vi "Earthquake.vi"(11 "VI Ref":refnum<vi>) -> ()   [LabVIEW 2019]
doc: "Earthquake disaster. Violently shakes the block diagram left and right, with each object having a 20% chance of being destroyed."
uses:
  _Sound/Music Player Command Message.ctl
  _Sound/Music Player Command.ctl
  _Sound/Sound.lvlib
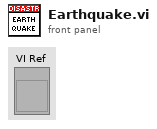
[diagram p1: front panel]
types:
  T1 = enum32{"Invalid", "Standard", "Closed", "Hidden", "Minimized", "Maximized"}
  T2 = typedef "Sound.lvlib/Music Player Command Message.ctl" = cluster{"Command":T3, "Data":variant}
  T3 = typedef "Sound.lvlib/Music Player Command.ctl" = enum16{"Enable", "Play", "Play Random", "Stop", "Shutdown"}
  T4 = typedef "LVPointTypeDef.ctl" = cluster{"Horizontal":i16, "Vertical":i16}
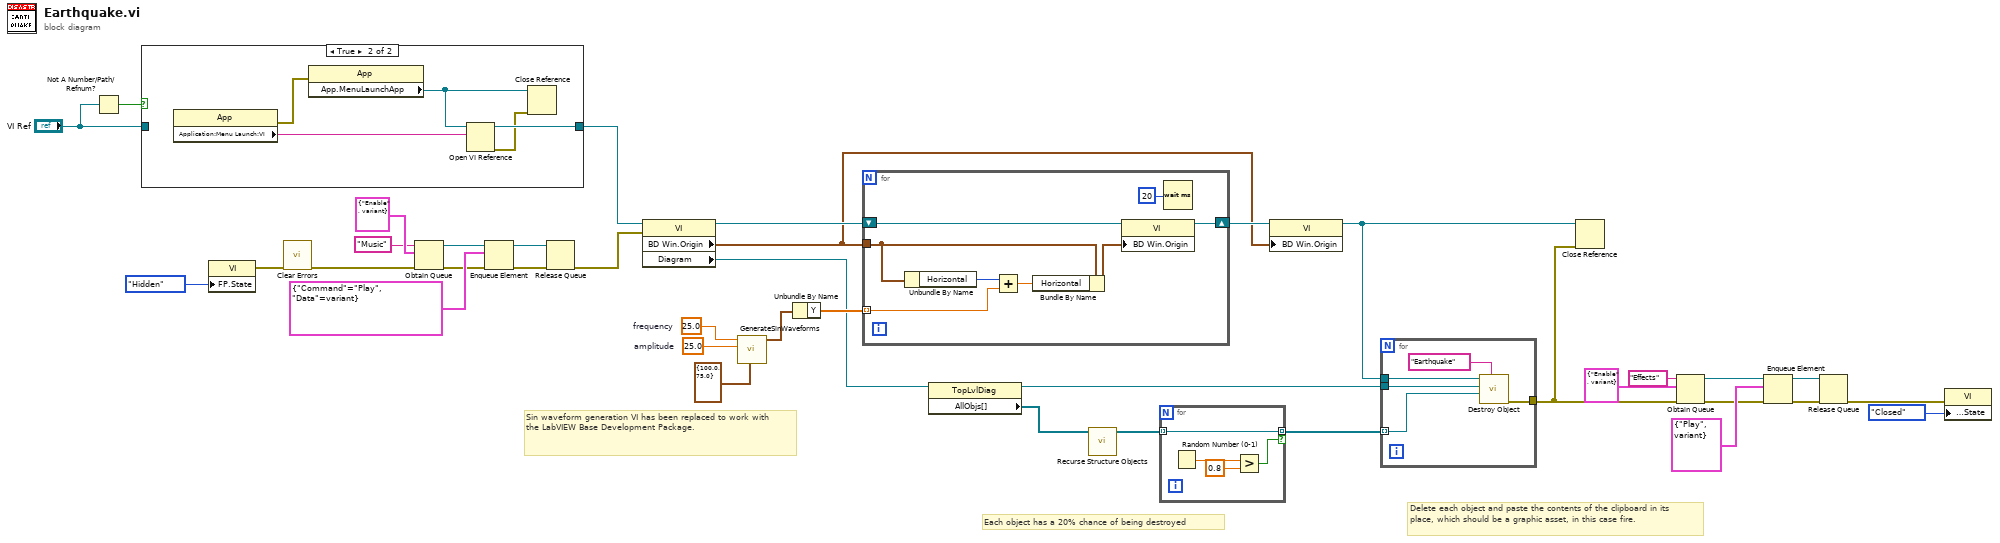
[diagram p0: block diagram]
diagram:
  w2 = 25.0  # amplitude
  w3 = 25.0  # frequency
  # "Sin waveform generation VI has been replaced to work with the LabVIEW Base Development Package."
  # "Delete each object and paste the contents of the clipboard in its place, which should be a graphic asset, in this case fire."
  # "Each object has a 20% chance of being destroyed"
  n1 = Not A Number/Path/Refnum?(number/path/refnum="VI Ref") -> (NaN/Path/Refnum?=w19:bool)
  n2 = case shown="True" w19 {
    tunnel: "VI Ref" -> [w39 _]
    tunnel: [w39 w43] -> w18
    frame False {
    }
    frame True {
      n3 = property class="App"() -> (error out=w42:errorcluster, "Application:Menu Launch:VI"=w44:string)  [unwired: 2 in, 1 out]
      n4 = property class="App"(error in=w42) -> ("App.MenuLaunchApp"=w40:refnum<vi>)  [unwired: 1 in, 2 out]
      n5 = Open VI Reference(application reference (local)=w40, vi path=w44) -> (vi reference=w43:refnum<vi>, error out=w41:errorcluster)  [unwired: 4 in]
      n6 = Close Reference(reference=w40, error in (no error)=w41) -> ()  [unwired: 1 out]
    }
  }
  n7 = property class="VI"("FP.State"=T1."Hidden" ("Front Panel Window:State")) -> (error out=w9:errorcluster)  [unwired: 2 in, 1 out]
  n8 = call <vilib>:"Clear Errors.vi"("error in (no error)"=w9) -> ("error out"=w8:errorcluster)  [unwired: 5 in, 1 out]
  n9 = Obtain Queue(name (unnamed)="Music", element data type=T2 {"Command"=enum."Enable", "Data"=variant} ("Message"), error in (no error)=w8) -> (queue out=w24:refnum<queue>, error out=w10:errorcluster)  [unwired: 2 in, 1 out]
  n10 = Enqueue Element(queue=w24, element=T2 {"Command"=enum."Play", "Data"=variant(string "Disasters\\Disaster Decision")}, error in (no error)=w10) -> (queue out=w23:refnum<queue>, error out=w22:errorcluster)  [unwired: 1 in, 1 out]
  n11 = Release Queue(queue=w23, error in (no error)=w22) -> (error out=w4:errorcluster)  [unwired: 1 in, 2 out]
  n12 = property class="VI"(reference=w18, error in=w4) -> (reference out=w38:refnum<vi>, "BD Win.Origin"=w36:T4, "Diagram"=w33:refnum<vi>)  [unwired: 1 out]
  n13 = call "GenerateSinWaveforms.vi"("sampling info"=cluster{"Fs":dbl, "#s":dbl} {"Fs"=100.0, "#s"=75.0}, "amplitude"=w2, "frequency"=w3) -> ("Waveform"=w35:waveform(dbl))  [unwired: 8 in]
  n14 = Unbundle By Name(w35) -> ("Y"=w34:dbl[])
  n15 = for {
    tunnel: w36 -> [w46]
    shift-right: [w47] -> w37
    shift-left: w38 -> [w52]
    tunnel: w34 -> [w45] mode=indexing
    n16 = Unbundle By Name(w46) -> ("Horizontal"=w51:i16)
    n17 = Add(x=w51, y=w45) -> (x+y=w50:dbl)
    n18 = Bundle By Name(cluster=w46, "Horizontal"=w50) -> (w49:T4)
    n19 = property class="VI"(reference=w52, "BD Win.Origin"=w49) -> (reference out=w47:refnum<vi>)  [unwired: 1 in, 1 out]
    n20 = Wait (ms)(milliseconds to wait=u32 20) -> ()  [unwired: 1 out]
  }
  n21 = property class="TopLvlDiag"(reference=w33) -> (reference out=w6:refnum<vi>, "AllObjs[]"=w14:refnum<vi>[])  [unwired: 1 in, 1 out]
  n22 = call "Recurse Structure Objects.vi"("Objects In"=w14) -> ("Objects Out"=w13:refnum<vi>[])  [unwired: 10 in]
  n23 = for {
    tunnel: w13 -> [w54] mode=indexing
    tunnel: [w54] -> w32 mode=indexing if=w53
    n24 = Random Number (0-1)() -> (number: 0 to 1=w56:dbl)
    n25 = Greater?(x=w56, y=0.8) -> (0:w53:bool)
  }
  n26 = property class="VI"(reference=w37, "BD Win.Origin"=w36) -> (reference out=w7:refnum<vi>)  [unwired: 1 in, 1 out]
  n27 = for {
    tunnel: w32 -> [w59] mode=indexing
    tunnel: w7 -> [w60]
    tunnel: w6 -> [w61]
    tunnel: [w57] -> w5
    n28 = call "Destroy Object.vi"("Undo Text"="Earthquake" ("Name"), "Object Ref"=w59, "BD Ref"=w61, "VI Ref"=w60) -> ("error out"=w57:errorcluster)  [unwired: 7 in]
  }
  n29 = Close Reference(reference=w7, error in (no error)=w5) -> ()  [unwired: 1 out]
  n30 = Obtain Queue(name (unnamed)="Effects", element data type=T2 {"Command"=enum."Enable", "Data"=variant} ("Message"), error in (no error)=w5) -> (queue out=w27:refnum<queue>, error out=w12:errorcluster)  [unwired: 2 in, 1 out]
  n31 = Enqueue Element(queue=w27, element=T2 {"Command"=enum."Play", "Data"=variant(string "siren")}, error in (no error)=w12) -> (queue out=w21:refnum<queue>, error out=w20:errorcluster)  [unwired: 1 in, 1 out]
  n32 = Release Queue(queue=w21, error in (no error)=w20) -> (error out=w15:errorcluster)  [unwired: 1 in, 2 out]
  n33 = property class="VI"(error in=w15, "Front Panel Window:State"=T1."Closed") -> ()  [unwired: 1 in, 2 out]
